vi "String Correct Whitespaces.vi"(11 "String in":string) -> (3 "String out":string)   [LabVIEW 2018]
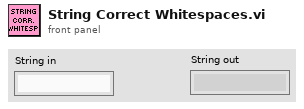
[diagram p1: front panel]
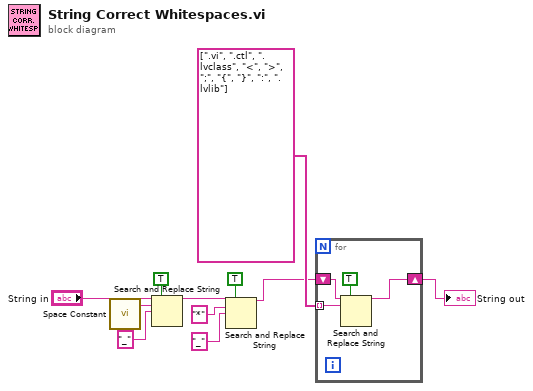
[diagram p0: block diagram]
diagram:
  n1 = call <vilib>:"Space Constant.vi"() -> ("String"=w10:string)
  n2 = Search and Replace String(replace all?=TRUE ("replace all? (F)"), input string="String in", search string=w10, replace string="_" ("replace string (\"\")")) -> (result string=w3:string)  [unwired: 4 in, 3 out]
  n3 = Search and Replace String(replace all?=TRUE ("replace all? (F)"), input string=w3, search string="*" ("replace string (\"\")"), replace string="_" ("replace string (\"\")")) -> (result string=w2:string)  [unwired: 4 in, 3 out]
  n4 = for {
    tunnel: string[] [".vi", ".ctl", ".lvclass", "<", ">", ";", "{", "}", ":", ".lvlib"] -> [w14] mode=indexing
    shift-right: [w12] -> w6
    shift-left: w2 -> [w13]
    n5 = Search and Replace String(replace all?=TRUE ("replace all? (F)"), input string=w13, search string=w14) -> (result string=w12:string)  [unwired: 5 in, 3 out]
  }
  "String out" <- w6
